vi "配置.vi"() -> (2 "启用参数":T1, 3 "串口输出":refnum<visa-resource-name>)   [LabVIEW 2016, in "斯坦道多参数.lvlib"]
uses:
  <vilib>/Utility/miscctls.llb/LVPointTypeDef.ctl
  <vilib>/Plasmionique/MB Master/MB_Master_Serial/MB_Master_Serial.lvclass
panel:
  in  "蓝绿藻":bool
  in  "关闭串口":bool
  in  "打开串口":bool
  in  "叶绿素a启用":bool
  in  "Temp":bool
  in  "Cond":bool
  in  "Turb":bool
  in  "DO":bool
  in  "pH":bool
  in  "关闭":bool
  in  "VISA资源名称":refnum<visa-resource-name>
  # "请设置串口参数"
  # "请选择要启用的参数"
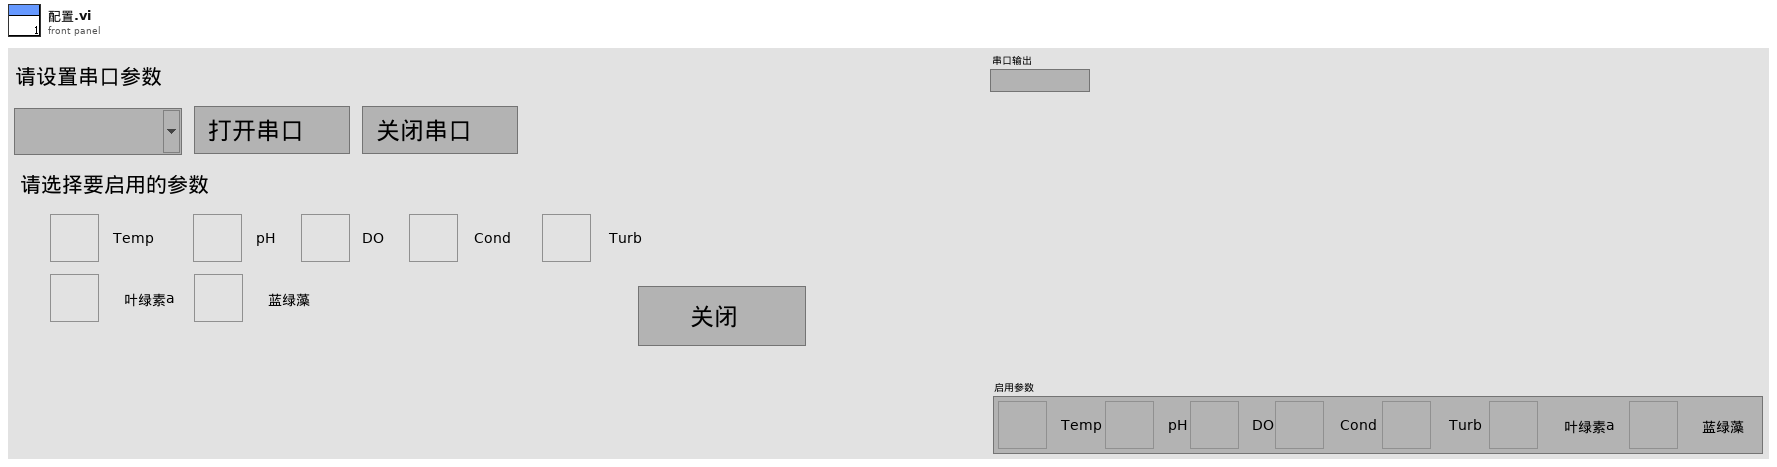
[diagram p1: front panel]
types:
  T1 = cluster{"Temp":bool, "pH":bool, "DO":bool, "Cond":bool, "Turb":bool, "叶绿素a启用":bool, "蓝绿藻":bool}
  T2 = typedef "LVPointTypeDef.ctl" = cluster{"Horizontal":i16, "Vertical":i16}
  T3 = enum8{"Enabled", "Disabled", "Disabled and Grayed Out"}
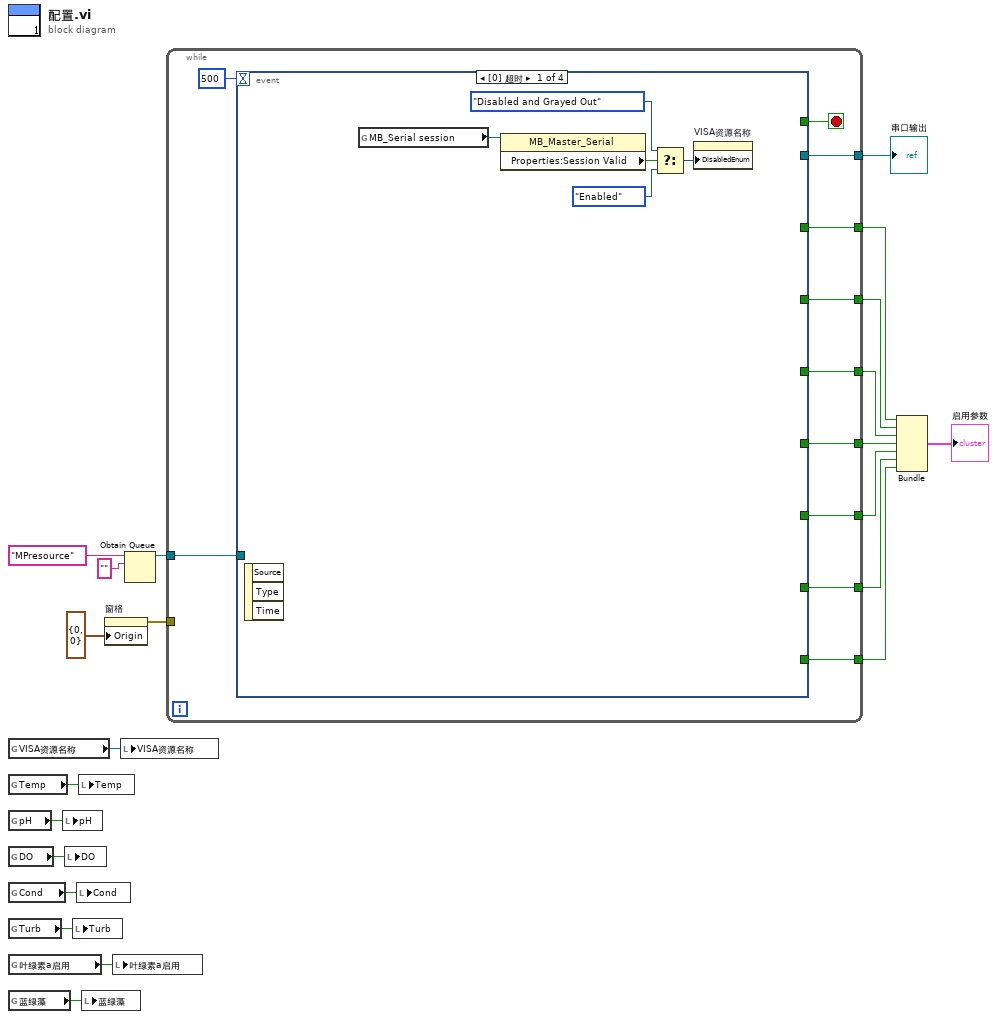
[diagram p0: block diagram]
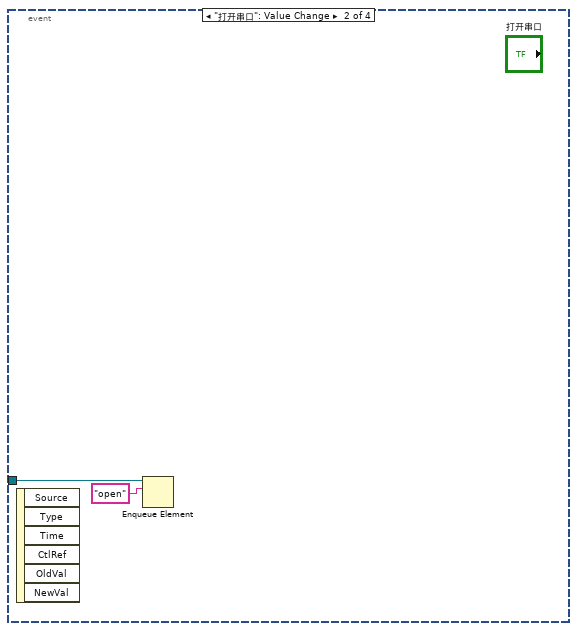
[diagram p2: hidden frame]
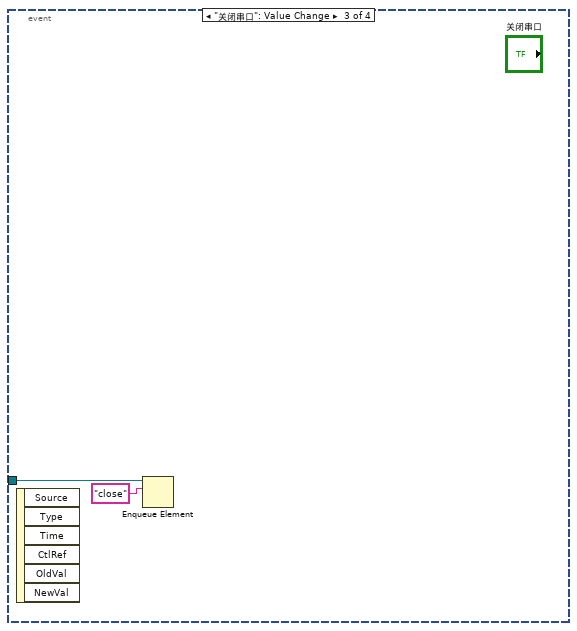
[diagram p3: hidden frame]
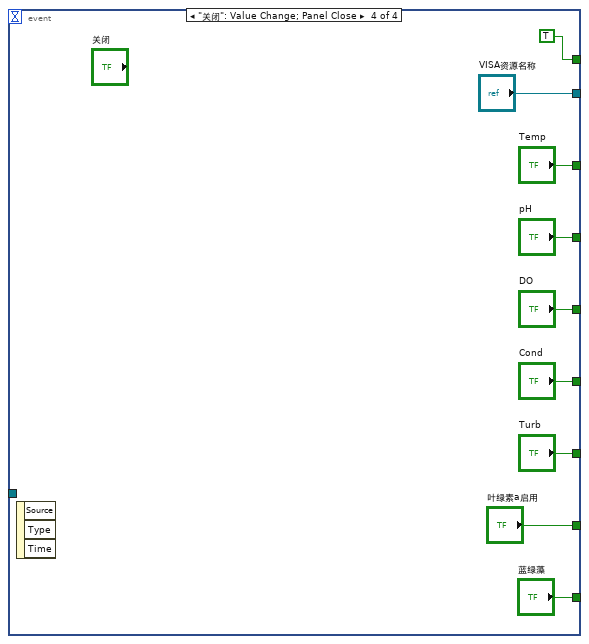
[diagram p4: hidden frame]
diagram:
  n1 = global read "断电保存变量.vi" "VISA资源名称"() -> (w15:refnum<visa-resource-name>)
  n2 = global read "断电保存变量.vi" "Temp"() -> (w10:bool)
  n3 = global read "断电保存变量.vi" "pH"() -> (w11:bool)
  n4 = global read "断电保存变量.vi" "DO"() -> (w12:bool)
  n5 = global read "断电保存变量.vi" "Cond"() -> (w13:bool)
  n6 = global read "断电保存变量.vi" "Turb"() -> (w14:bool)
  n7 = global read "断电保存变量.vi" "叶绿素a启用"() -> (w6:bool)
  n8 = global read "断电保存变量.vi" "蓝绿藻"() -> (w1:bool)
  n9 = local write "pH"(w11) -> ()
  n10 = local write "DO"(w12) -> ()
  n11 = local write "Turb"(w14) -> ()
  n12 = local write "Cond"(w13) -> ()
  n13 = local write "Temp"(w10) -> ()
  n14 = local write "蓝绿藻"(w1) -> ()
  n15 = property on="窗格" class="Pane"("Origin"=T2 {"Horizontal"=0, "Vertical"=0} ("原点")) -> (error out=w8:errorcluster)  [unwired: 2 in, 1 out]
  n16 = local write "叶绿素a启用"(w6) -> ()
  n17 = local write "VISA资源名称"(w15) -> ()
  n18 = Obtain Queue(name (unnamed)="MPresource" ("名称（未命名）"), element data type="" ("名称（未命名）")) -> (queue out=w3:refnum<queue>)  [unwired: 3 in, 2 out]
  n19 = while {
    tunnel: [w32] -> w22
    tunnel: [w31] -> w21
    tunnel: [w30] -> w20
    tunnel: [w29] -> w19
    tunnel: [w28] -> w18
    tunnel: [w27] -> w17
    tunnel: [w26] -> w9
    tunnel: w8 -> [_]
    tunnel: w3 -> [w25]
    tunnel: [w24] -> w2
    stop <- w33 stop-if-true
    n20 = event shown="[0] 超时" {
      selector: _ -> [_ _ _ _]
      dyn-events: _ -> [_ _ _ _]
      timeout: 500 -> [_ _ _ _]
      tunnel: [_ _ _ TRUE] -> w33
      tunnel: [_ _ _ "VISA资源名称"] -> w32
      tunnel: [_ _ _ "Temp"] -> w31
      tunnel: [_ _ _ "pH"] -> w30
      tunnel: [_ _ _ "DO"] -> w29
      tunnel: [_ _ _ "Cond"] -> w28
      tunnel: [_ _ _ "Turb"] -> w27
      tunnel: [_ _ _ "叶绿素a启用"] -> w26
      tunnel: w25 -> [_ w40 w42 _]
      tunnel: [_ _ _ "蓝绿藻"] -> w24
      event Timeout {
        n21 = event-data() -> ()  [unwired: 1 in, 3 out]
        n22 = global read "多参数全局变量.vi" "MB_Serial session"() -> (w38:refnum<class "MB_Master_Serial.lvclass">)
        n23 = property class="MB_Master_Serial"(reference=w38) -> ("Properties:Session Valid"=w37:bool)  [unwired: 1 in, 2 out]
        n24 = Select(t=T3."Disabled and Grayed Out" ("禁用"), s=w37, f=T3."Enabled" ("禁用")) -> (s? t:f=w34:T3)
        n25 = property on="VISA资源名称" class="VISAName"("DisabledEnum"=w34) -> ()  [unwired: 2 in, 2 out]
      }
      event "打开串口": Value Change {
        n26 = event-data() -> ()  [unwired: 1 in, 6 out]
        n27 = Enqueue Element(queue=w40, element="open" ("元素")) -> ()  [unwired: 2 in, 3 out]
      }
      event "关闭串口": Value Change {
        n28 = event-data() -> ()  [unwired: 1 in, 6 out]
        n29 = Enqueue Element(queue=w42, element="close" ("元素")) -> ()  [unwired: 2 in, 3 out]
      }
      event "关闭": Value Change; Panel Close {
        n30 = event-data() -> ()  [unwired: 1 in, 3 out]
      }
    }
  }
  "串口输出" <- w22
  n31 = Bundle("Temp"=w21, "pH"=w20, "DO"=w19, "Cond"=w18, "Turb"=w17, "叶绿素a启用"=w9, "蓝绿藻"=w2) -> (→"启用参数":T1)  [unwired: 1 in]
